vi "Target Groups.vi"(8 "error in (no error)":errorcluster, 11 "Cluster in":refnum<class "Cluster Config.lvclass">) -> (0 "error out":errorcluster, 2 "Target Groups":T1[](array[typedef]), 3 "Cluster out":refnum<class "Cluster Config.lvclass">)   [LabVIEW 2020, in "VolatusConfig.lvlib" / "Cluster Config.lvclass"]
uses:
  Cluster Config.lvclass
  C:/dev/lv20CE/relink/lv-volatus/VolatusConfig/VolatusConfigElement/VolatusConfigElement.lvclass
  Target Group.ctl
  VolatusConfigElement/VolatusConfigElement.lvclass/VolatusConfigElement.ctl
  VolatusConfigElement/Element.vi
  Cluster Config.lvclass/Cluster Config.ctl
  VolatusConfigElement/VolatusConfigElement.lvclass
  lv-cdm/CDM-Config/Config Element/Config Element.lvclass
  VolatusConfig.lvlib
  C:/dev/lv20CE/relink/lv-volatus/VolatusConfig/Cluster/Cluster Config.lvclass
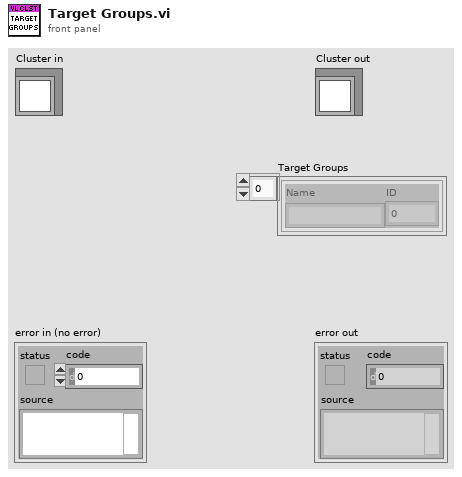
[diagram p1: front panel]
types:
  T1 = typedef "VolatusConfig.lvlib/Target Group.ctl" = cluster{"Name":string, "ID":u32}
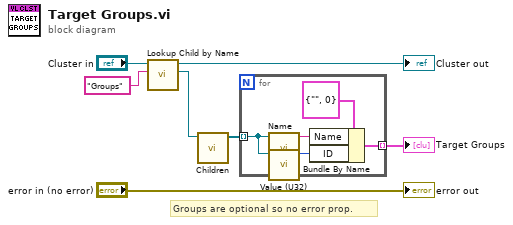
[diagram p0: block diagram]
diagram:
  # "Groups are optional so no error prop."
  n1 = call "Lookup Child by Name.vi"("Child Name"="Groups", "VolatusConfigElement in"="Cluster in") -> ("Child"=w3:refnum<class "Config Element.lvclass">, "VolatusConfigElement out"=→"Cluster out":refnum<class "Cluster Config.lvclass">)  [unwired: 6 in, 2 out]
  n2 = call "Children.vi"("Config Element in"=w3) -> ("Elements"=w4:refnum<class "Config Element.lvclass">[])  [unwired: 9 in, 1 out]
  n3 = for {
    tunnel: w4 -> [w12] mode=indexing
    tunnel: [w8] -> w2 mode=indexing
    n4 = call "Name.vi"("Config Element in"=w12) -> ("Name"=w10:string)  [unwired: 9 in, 1 out]
    n5 = call "Value (U32).vi"("Config Element in"=w12) -> ("U32 Value"=w9:u32)  [unwired: 9 in, 1 out]
    n6 = Bundle By Name(cluster=T1 {"Name"="", "ID"=0} ("Target Group"), "Name"=w10, "ID"=w9) -> (w8:T1)
  }
  "Target Groups" <- w2
  "error out" <- "error in (no error)"
